vi "ABR3-Estimate Threshold.vi"(0 "Level (in)":dbl[](array[numeric]), 5 "Neural":dbl[][](array[numeric]), 7 "dt (us)":dbl, 9 "Threshold Estimation":T3={"Tmin (ms)"=1.0, "Tmax (ms)"=6.0, "CC criterion"=0.35, "adjR2 criterion"=0.0}, 11 "error in (no error)":errorcluster) -> (8 "Threshold":dbl, 10 "Work":T1, 15 "error out":errorcluster)   [LabVIEW 2020]
uses:
  ABR3-Threshold Estimation Parameters.ctl
  ABR3-Threshold Estimation Work.ctl
  ABR3-Threshold Estimation Result.ctl
panel:
  out "Logistic":string
  out "Power2":string
  out "Graph":cluster{dbl[], dbl[]}[](graph)
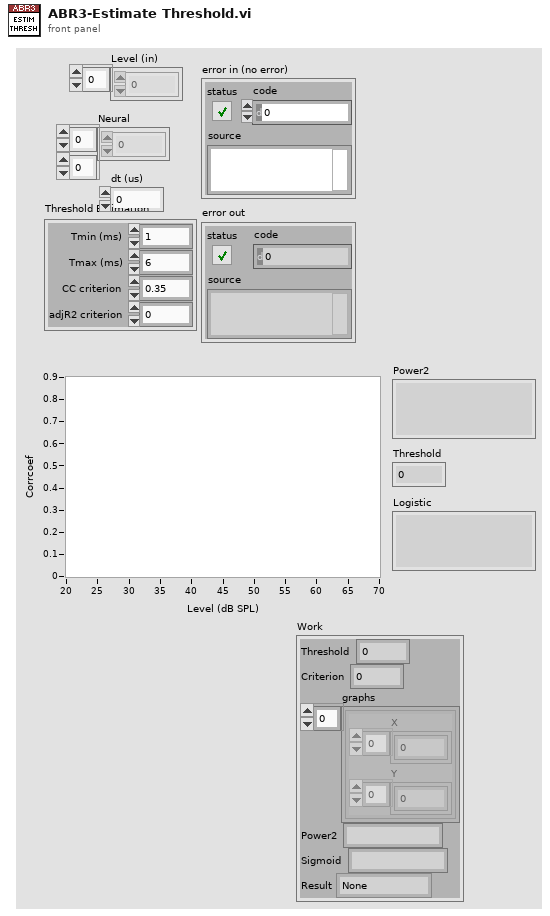
[diagram p1: front panel]
types:
  T1 = typedef "ABR3-Threshold Estimation Work.ctl" = cluster{"Threshold":dbl, "Criterion":dbl, "graphs":cluster{"X":dbl[], "Y":dbl[]}[], "Power2":string, "Sigmoid":string, "Result":T2}
  T2 = typedef "ABR3-Threshold Estimation Result.ctl" = enum16{"None", "Power", "Sigmoid", "Power (noisy)", "Suprathreshold", "Invalid"}
  T3 = typedef "ABR3-Threshold Estimation Parameters.ctl" = cluster{"Tmin (ms)":dbl, "Tmax (ms)":dbl, "CC criterion":dbl, "adjR2 criterion":dbl}
  T4 = cluster{"positive x":dbl[], "best nonlinear fit":dbl[]}
  T5 = cluster{"Level (out)":dbl[], "best nonlinear fit":dbl[]}
  T6 = cluster{"Level (out)":dbl[], "best nonlinear fit":dbl[]}[]
  T7 = cluster{"X":dbl, "CC criterion":dbl, cluster{"Level (out)":dbl[], "best nonlinear fit":dbl[]}[], "summary":string, "summary":string, "Result":T2}
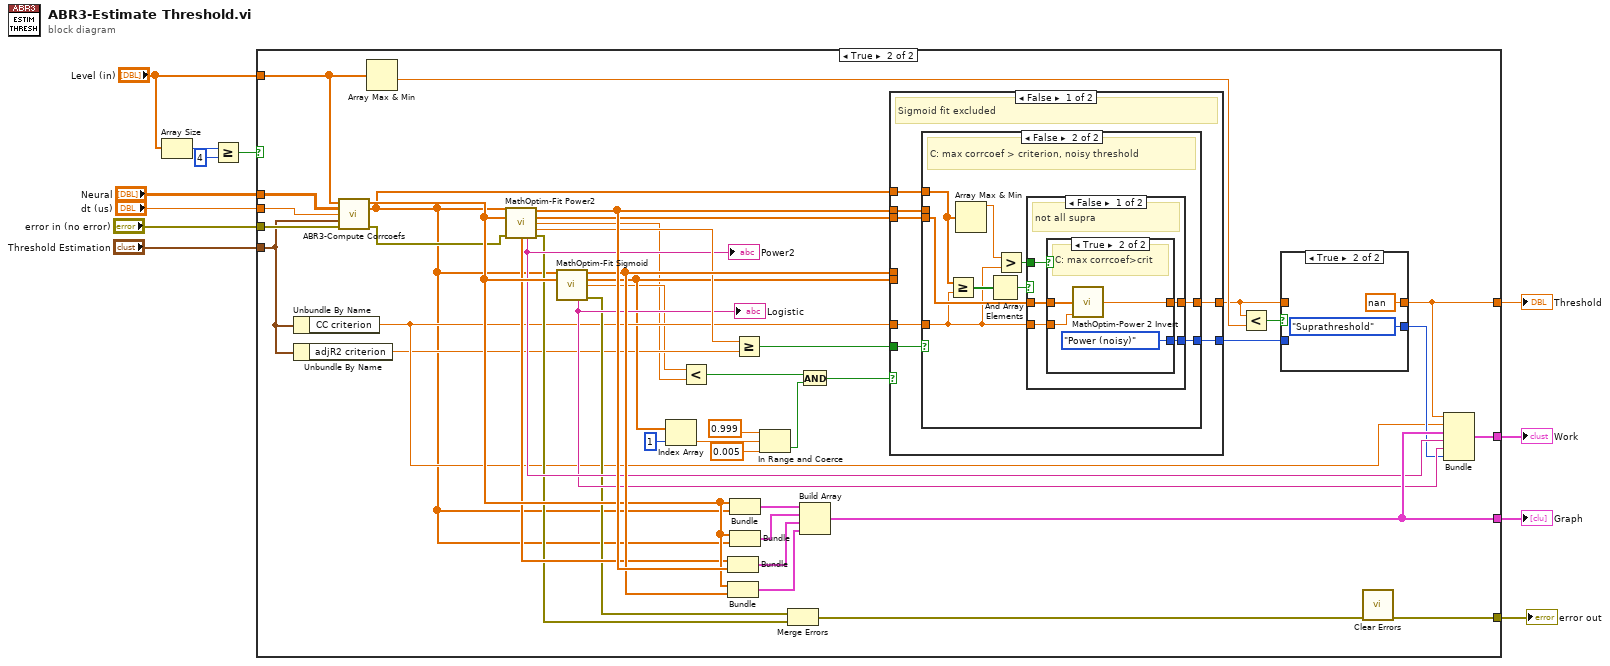
[diagram p0: block diagram]
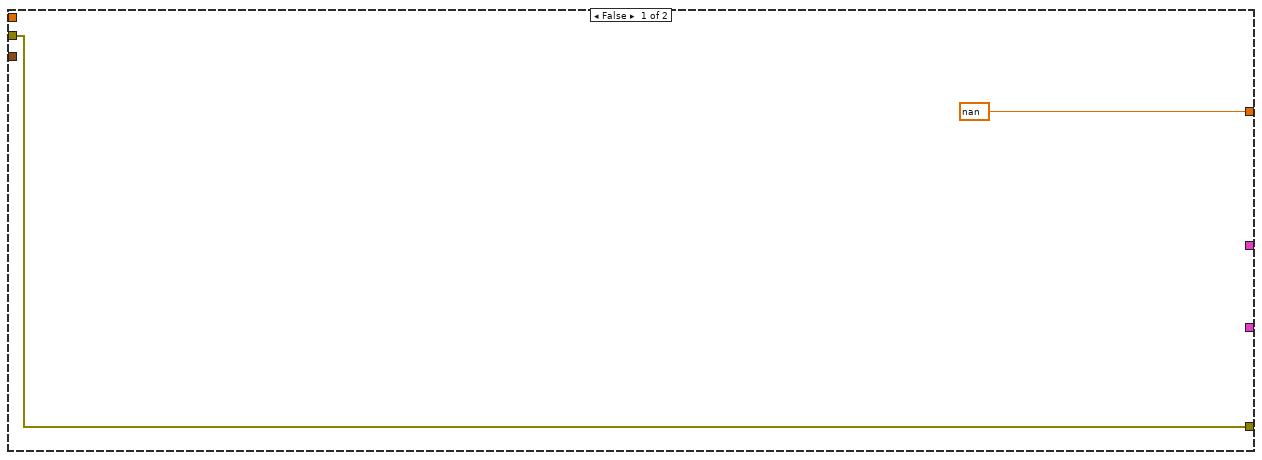
[diagram p2: hidden frame]
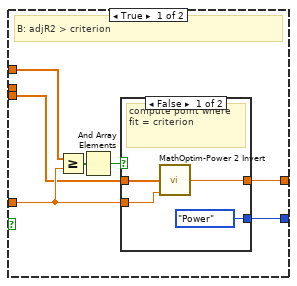
[diagram p4: hidden frame]
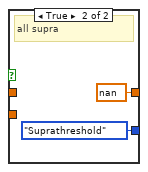
[diagram p5: hidden frame]
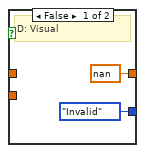
[diagram p6: hidden frame]
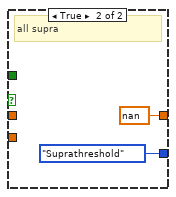
[diagram p7: hidden frame]
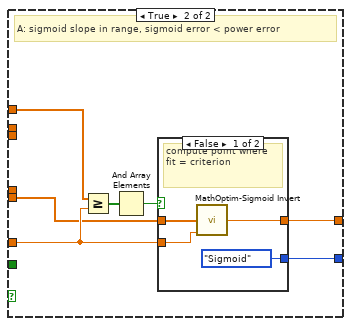
[diagram p8: hidden frame]
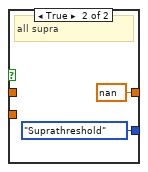
[diagram p9: hidden frame]
diagram:
  n1 = Array Size(array="Level (in)") -> (size(s)=w4:i32)
  n2 = Greater Or Equal?(x=w4, y=4) -> (x >= y?=w3:bool)
  n3 = case shown="True" w3 {
    tunnel: "error in (no error)" -> [w13 w54]
    tunnel: "Threshold Estimation" -> [_ w22]
    tunnel: "Level (in)" -> [_ w33]
    tunnel: "Neural" -> [_ w47]
    tunnel: "dt (us)" -> [_ w46]
    tunnel: [nan ("X") w29] -> w8
    tunnel: [_ w45] -> w7
    tunnel: [_ w44] -> w6
    tunnel: [w13 w37] -> w1
    frame False {
    }
    frame True {
      n4 = Unbundle By Name(w22) -> ("CC criterion"=w26:dbl)
      n5 = Unbundle By Name(w22) -> ("adjR2 criterion"=w21:dbl)
      n6 = call "ABR3-Compute Corrcoefs.vi"("Level (in)"=w33, "Neural"=w47, "dt (us)"=w46, "Threshold Estimation"=w22, "error in (no error)"=w54) -> ("Level (out)"=w49:dbl[], "Corrcoefs"=w15:dbl[], "error out"=w48:errorcluster)  [unwired: 8 in]
      n7 = Array Max & Min(array=w33) -> (min value=w32:dbl)  [unwired: 3 out]
      n8 = call "MathOptim-Fit Power2.vi"("Y"=w15, "X"=w49, "error in (no error)"=w48) -> ("best nonlinear fit"=w53:dbl[], "best fit parameters"=w50:dbl[], "SSE"=w19:dbl, "adjusted R2"=w51:dbl, "positive x"=w41:dbl[], "summary"=w43:string, "error out"=w38:errorcluster)  [unwired: 6 in]
      "Power2" <- w43
      n9 = call "MathOptim-Fit Sigmoid.vi"("Y"=w15, "X"=w49) -> ("best nonlinear fit"=w52:dbl[], "best fit parameters"=w25:dbl[], "SSE"=w20:dbl, "summary"=w42:string, "error out"=w40:errorcluster)  [unwired: 8 in, 1 out]
      "Logistic" <- w42
      n10 = Index Array(array=w25, index=1) -> (element=w24:dbl)
      n11 = Less?(x=w20, y=w19) -> (x < y?=w18:bool)
      n12 = Bundle("positive x"=w41, "best nonlinear fit"=w53) -> (w56:T4)  [unwired: 1 in]
      n13 = Bundle("Level (out)"=w49, "best nonlinear fit"=w52) -> (w55:T5)  [unwired: 1 in]
      n14 = Bundle("Level (out)"=w49, "Corrcoefs"=w15) -> (w58:cluster{"Level (out)":dbl[], "Corrcoefs":dbl[]})  [unwired: 1 in]
      n15 = Bundle("Level (out)"=w49, "Corrcoefs"=w15) -> (w57:cluster{"Level (out)":dbl[], "Corrcoefs":dbl[]})  [unwired: 1 in]
      n16 = Greater Or Equal?(x=w51, y=w21) -> (x >= y?=w16:bool)
      n17 = In Range and Coerce(upper limit=0.999, x=w24, lower limit=0.005) -> (In Range?=w34:bool)  [unwired: 1 out]
      n18 = Merge Errors(w40, w38) -> (w39:errorcluster)
      n19 = And(x=w18, y=w34) -> (x .and. y?=w17:bool)
      n20 = Build Array(w58, w57, w56, w55) -> (w45:T6)
      n21 = case shown="False" w17 {
        tunnel: w53 -> [w67 _]
        tunnel: w52 -> [_ _]
        tunnel: w26 -> [w66 w111]
        tunnel: w50 -> [w68 _]
        tunnel: w25 -> [_ w110]
        tunnel: [w63 w109] -> w30
        tunnel: [w64 w108] -> w27
        tunnel: w15 -> [w65 w106]
        tunnel: w16 -> [w69 _]
        frame False {
          # "Sigmoid fit excluded"
          n22 = case shown="False" w69 {
            tunnel: w67 -> [_ _]
            tunnel: w66 -> [w73 w84]
            tunnel: w68 -> [w71 w90]
            tunnel: [w76 w89] -> w63
            tunnel: [w75 w88] -> w64
            tunnel: w65 -> [w72 w85]
            frame True {
              # "B: adjR2 > criterion"
              n23 = Greater Or Equal?(x=w72, y=w73) -> (x >= y?=w74:bool[])
              n24 = And Array Elements(Boolean array=w74) -> (logical AND=w70:bool)
              n25 = case shown="False" w70 {
                tunnel: w73 -> [w79 _]
                tunnel: w71 -> [w80 _]
                tunnel: [w78 nan ("X")] -> w76
                tunnel: [ABR3-Threshold_Estimation_Result."Power" ("Result") ABR3-Threshold_Estimation_Result."Suprathreshold" ("Result")] -> w75
                frame False {
                  # "compute point where\nfit = criterion"
                  n26 = call "MathOptim-Power 2 Invert.vi"("Parameters"=w80, "Y"=w79) -> ("X"=w78:dbl)  [unwired: 13 in]
                }
                frame True {
                  # "all supra"
                }
              }
            }
            frame False {
              # "C: max corrcoef > criterion, noisy threshold"
              n27 = Greater Or Equal?(x=w85, y=w84) -> (x >= y?=w87:bool[])
              n28 = Array Max & Min(array=w85) -> (max value=w83:dbl)  [unwired: 3 out]
              n29 = And Array Elements(Boolean array=w87) -> (logical AND=w86:bool)
              n30 = Greater?(x=w83, y=w84) -> (0:w91:bool)
              n31 = case shown="False" w86 {
                tunnel: w84 -> [w95 _]
                tunnel: w90 -> [w96 _]
                tunnel: [w94 nan ("X")] -> w89
                tunnel: [w93 ABR3-Threshold_Estimation_Result."Suprathreshold" ("Result")] -> w88
                tunnel: w91 -> [w92 _]
                frame False {
                  # "not all supra"
                  n32 = case shown="True" w92 {
                    tunnel: w96 -> [_ w102]
                    tunnel: w95 -> [_ w101]
                    tunnel: [nan ("X") w100] -> w94
                    tunnel: [ABR3-Threshold_Estimation_Result."Invalid" ("Result") ABR3-Threshold_Estimation_Result."Power (noisy)" ("Result")] -> w93
                    frame False {
                      # "D: Visual"
                    }
                    frame True {
                      # "C: max corrcoef>crit"
                      n33 = call "MathOptim-Power 2 Invert.vi"("Parameters"=w102, "Y"=w101) -> ("X"=w100:dbl)  [unwired: 13 in]
                    }
                  }
                }
                frame True {
                  # "all supra"
                }
              }
            }
          }
        }
        frame True {
          # "A: sigmoid slope in range, sigmoid error < power error"
          n34 = Greater Or Equal?(x=w106, y=w111) -> (x >= y?=w107:bool[])
          n35 = And Array Elements(Boolean array=w107) -> (logical AND=w105:bool)
          n36 = case shown="False" w105 {
            tunnel: w111 -> [w114 _]
            tunnel: w110 -> [w115 _]
            tunnel: [w113 nan ("X")] -> w109
            tunnel: [ABR3-Threshold_Estimation_Result."Sigmoid" ("Result") ABR3-Threshold_Estimation_Result."Suprathreshold" ("Result")] -> w108
            frame False {
              # "compute point where\nfit = criterion"
              n37 = call "MathOptim-Sigmoid Invert.vi"("Parameters"=w115, "Y"=w114) -> ("X"=w113:dbl)  [unwired: 13 in]
            }
            frame True {
              # "all supra"
            }
          }
        }
      }
      n38 = Less?(x=w30, y=w32) -> (x < y?=w31:bool)
      n39 = case shown="True" w31 {
        tunnel: w30 -> [w60 _]
        tunnel: [w60 nan] -> w29
        tunnel: [w59 ABR3-Threshold_Estimation_Result."Suprathreshold" ("Result")] -> w28
        tunnel: w27 -> [w59 _]
        frame False {
        }
        frame True {
        }
      }
      n40 = call <vilib>:"Clear Errors.vi"("error in (no error)"=w39) -> ("error out"=w37:errorcluster)  [unwired: 5 in, 1 out]
      n41 = Bundle("X"=w29, "CC criterion"=w26, w45, "summary"=w43, "summary"=w42, "Result"=w28) -> (w44:T7)  [unwired: 1 in]
    }
  }
  "Graph" <- w7
  "Threshold" <- w8
  "Work" <- w6
  "error out" <- w1
